vi "setNSteps.vi"(7 "FWD":bool=TRUE, 8 "error in":errorcluster, 9 "setnSteps in":dbl, 10 "axis in":u8, 11 "connection ID":refnum<k5>) -> (0 "error out":errorcluster, 1 "setnSteps out":dbl, 2 "axis out":u8, 3 "connection ID":refnum<k5>)   [LabVIEW 2016]
panel:
  in  "Set Command":string="com.attocube.amc.move.setNSteps"
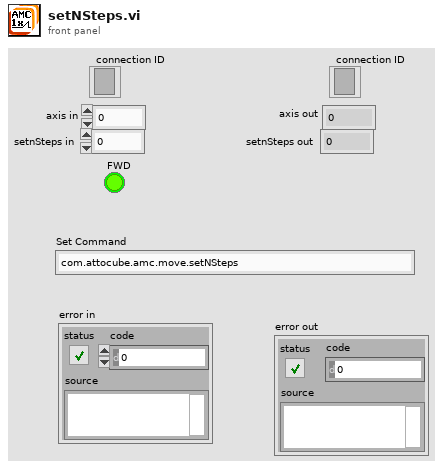
[diagram p1: front panel]
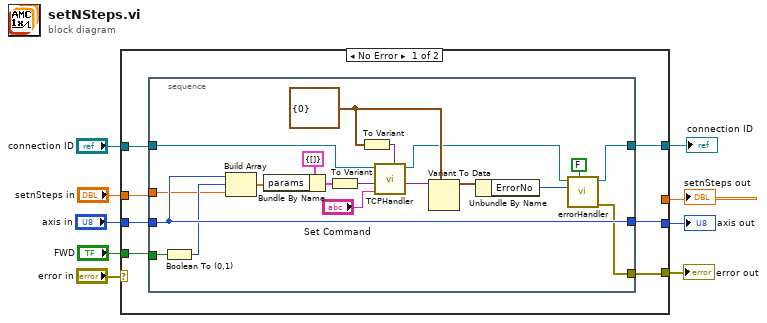
[diagram p0: block diagram]
diagram:
  n1 = case shown="No Error" "error in" {
    selector: "error in" -> [_ w36]
    tunnel: "axis in" -> [w14 w39]
    tunnel: [w10 w36] -> w8
    tunnel: [w11 w39] -> w7
    tunnel: "setnSteps in" -> [w16 w38]
    tunnel: [w12 w37] -> w5
    tunnel: "connection ID" -> [w13 w37]
    tunnel: "FWD" -> [w15 _]
    tunnel: [_ w38] -> w1
    frame No Error {
      n2 = stacked-sequence {
        tunnel: [w17] -> w12
        tunnel: w13 -> [w25]
        tunnel: w14 -> [w27]
        tunnel: [w27] -> w11
        tunnel: [w26] -> w10
        tunnel: w15 -> [w21]
        tunnel: w16 -> [w19]
        frame #0 {
          w23 = cluster{"ErrorNo":i64} {"ErrorNo"=0} ("input cluster")
          n3 = Boolean To (0,1)(Boolean=w21) -> (0, 1=w20:i16)
          n4 = Build Array(w27, w20, w19) -> (w31:dbl[])
          n5 = Bundle By Name(cluster=cluster{"params":i32[]} {"params"=[]} ("input cluster"), "params"=w31) -> (w32:cluster{"params":i32[]})
          n6 = To Variant(anything=w32) -> (Variant=w33:variant)
          n7 = To Variant(anything=w23) -> (Variant=w24:variant)
          n8 = call "TCPHandler.vi"("result Types"=w24, "method"="Set Command", "params"=w33, "connection ID"=w25) -> ("result"=w29:variant, "connection ID"=w18:refnum<k5>)  [unwired: 5 in, 1 out]
          n9 = Variant To Data(type=w23, Variant=w29) -> (data=w34:cluster{"ErrorNo":i64})  [unwired: 1 in, 1 out]
          n10 = Unbundle By Name(w34) -> ("ErrorNo"=w35:i64)
          n11 = call "errorHandler.vi"("show popup"=FALSE, "error number"=w35, "connection ID"=w18) -> ("error out"=w26:errorcluster, "connection ID"=w17:refnum<k5>)  [unwired: 7 in]
        }
      }
    }
    frame Error {
    }
  }
  "error out" <- w8
  "axis out" <- w7
  "setnSteps out" <- w1
  "connection ID" <- w5
